vi "nanocal -- nuclear schottky fit V4.vi"() -> ()   [LabVIEW 2020] (continued)
  out "string OUT":string="  \"IDS0158_210310_RAW_cal__ref_\" ->   <| \"ζ\"->  0.331549170129  , \"τ1\"-> 0.031957261989  , \"τS\"-> 0.245155954508  , \"τN\"-> 0.327332604975  , \"τC\"-> 0.001044440547  , \"κ0\"-> 0.000000000511  , \"mm1\"-> 0.000000000000  , \"mm2\"-> 0.000000000000  , \"mm3\"-> 0.000000000000  , \"T\"->  0.140000000000  , \"B\"-> 12.000000000000  , \"θ\"-> 0.000000000000  |>   , \r\"IDS0158_210310_RAW_cal__sam_\" ->   <| \"ζ\"->  0.286336668596  , \"τ1\"-> 0.037477267671  , \"τS\"-> 0.354459287884  , \"τN\"-> 0.444916383639  , \"τC\"-> 0.001225600579  , \"κ0\"-> 0.000000000596  , \"mm1\"-> 0.000000000000  , \"mm2\"-> 0.000000000000  , \"mm3\"-> 0.000000000000  , \"T\"->  0.140000000000  , \"B\"-> 12.000000000000  , \"θ\"-> 0.000000000000  |>   , \r\"IDS0159_210310_RAW_cal__ref_\" ->   <| \"ζ\"->  0.269623663752  , \"τ1\"-> 0.029946823009  , \"τS\"-> 0.193020268264  , \"τN\"-> 0.181925572107  , \"τC\"-> 0.001029221853  , \"κ0\"-> 0.000000000645  , \"mm1\"-> 0.000000000000  , \"mm2\"-> 0.000000000000  , \"mm3\"-> 0.000000000000  , \"T\"->  0.170000000000  , \"B\"-> 12.000000000000  , \"θ\"-> 0.000000000000  |>   , \r\"IDS0159_210310_RAW_cal__sam_\" ->   <| \"ζ\"->  0.219100303741  , \"τ1\"-> 0.028643012604  , \"τS\"-> 0.279362928811  , \"τN\"-> 0.246156444058  , \"τC\"-> 0.001272401549  , \"κ0\"-> 0.000000000760  , \"mm1\"-> 0.000000000000  , \"mm2\"-> 0.000000000000  , \"mm3\"-> 0.000000000000  , \"T\"->  0.170000000000  , \"B\"-> 12.000000000000  , \"θ\"-> 0.000000000000  |>   , \r\"IDS0160_210310_RAW_cal__ref_\" ->   <| \"ζ\"->  0.207047266456  , \"τ1\"-> 0.027475093360  , \"τS\"-> 0.117497913331  , \"τN\"-> 0.102020652890  , \"τC\"-> 0.000950950989  , \"κ0\"-> 0.000000000918  , \"mm1\"-> 0.000000000000  , \"mm2\"-> 0.000000000000  , \"mm3\"-> 0.000000000000  , \"T\"->  0.200000000000  , \"B\"-> 12.000000000000  , \"θ\"-> 0.000000000000  |>   , \r\"IDS0160_210310_RAW_cal__sam_\" ->   <| \"ζ\"->  0.170488637524  , \"τ1\"-> 0.029234231120  , \"τS\"-> 0.149095458227  , \"τN\"-> 0.151792620275  , \"τC\"-> 0.001113424175  , \"κ0\"-> 0.000000001042  , \"mm1\"-> 0.000000000000  , \"mm2\"-> 0.000000000000  , \"mm3\"-> 0.000000000000  , \"T\"->  0.200000000000  , \"B\"-> 12.000000000000  , \"θ\"-> 0.000000000000  |>   , \r\"IDS0161_210310_RAW_cal__ref_\" ->   <| \"ζ\"->  0.165418845287  , \"τ1\"-> 0.025256902580  , \"τS\"-> 0.095232124148  , \"τN\"-> 0.068477414693  , \"τC\"-> 0.001100413424  , \"κ0\"-> 0.000000001058  , \"mm1\"-> 0.000000000000  , \"mm2\"-> 0.000000000000  , \"mm3\"-> 0.000000000000  , \"T\"->  0.220000000000  , \"B\"-> 12.000000000000  , \"θ\"-> 0.000000000000  |>   , \r\"IDS0161_210310_RAW_cal__sam_\" ->   <| \"ζ\"->  0.130531197151  , \"τ1\"-> 0.025704482770  , \"τS\"-> 0.129606657196  , \"τN\"-> 0.091602369165  , \"τC\"-> 0.001441379995  , \"κ0\"-> 0.000000001211  , \"mm1\"-> 0.000000000000  , \"mm2\"-> 0.000000000000  , \"mm3\"-> 0.000000000000  , \"T\"->  0.220000000000  , \"B\"-> 12.000000000000  , \"θ\"-> 0.000000000000  |>   , \r\"IDS0162_210310_RAW_cal__ref_\" ->   <| \"ζ\"->  0.094488415983  , \"τ1\"-> 0.023440091411  , \"τS\"-> 0.070629137621  , \"τN\"-> 0.023695223047  , \"τC\"-> 0.001462465509  , \"κ0\"-> 0.000000001371  , \"mm1\"-> 0.000000000000  , \"mm2\"-> 0.000000000000  , \"mm3\"-> 0.000000000000  , \"T\"->  0.280000000000  , \"B\"-> 12.000000000000  , \"θ\"-> 0.000000000000  |>   , \r\"IDS0162_210310_RAW_cal__sam_\" ->   <| \"ζ\"->  0.078258046754  , \"τ1\"-> 0.028009840731  , \"τS\"-> 0.092122038762  , \"τN\"-> 0.030129595899  , \"τC\"-> 0.001641062244  , \"κ0\"-> 0.000000001543  , \"mm1\"-> 0.000000000000  , \"mm2\"-> 0.000000000000  , \"mm3\"-> 0.000000000000  , \"T\"->  0.280000000000  , \"B\"-> 12.000000000000  , \"θ\"-> 0.000000000000  |>   , \r\"IDS0163_210310_RAW_cal__ref_\" ->   <| \"ζ\"->  0.066045279838  , \"τ1\"-> 0.021690723483  , \"τS\"-> 0.054398710223  , \"τN\"-> 0.012159058060  , \"τC\"-> 0.001677829713  , \"κ0\"-> 0.000000001745  , \"mm1\"-> 0.000000000000  , \"mm2\"-> 0.000000000000  , \"mm3\"-> 0.000000000000  , \"T\"->  0.330000000000  , \"B\"-> 12.000000000000  , \"θ\"-> 0.000000000000  |>   , \r\"IDS0163_210310_RAW_cal__sam_\" ->   <| \"ζ\"->  0.054088186012  , \"τ1\"-> 0.023838802615  , \"τS\"-> 0.069079396629  , \"τN\"-> 0.016435267456  , \"τC\"-> 0.002025071743  , \"κ0\"-> 0.000000001955  , \"mm1\"-> 0.000000000000  , \"mm2\"-> 0.000000000000  , \"mm3\"-> 0.000000000000  , \"T\"->  0.330000000000  , \"B\"-> 12.000000000000  , \"θ\"-> 0.000000000000  |>   , \r\"IDS0164_210310_RAW_cal__ref_\" ->   <| \"ζ\"->  0.046429657722  , \"τ1\"-> 0.021005913305  , \"τS\"-> 0.044250298502  , \"τN\"-> 0.006399419767  , \"τC\"-> 0.002349605146  , \"κ0\"-> 0.000000002166  , \"mm1\"-> 0.000000000000  , \"mm2\"-> 0.000000000000  , \"mm3\"-> 0.000000000000  , \"T\"->  0.400000000000  , \"B\"-> 12.000000000000  , \"θ\"-> 0.000000000000  |>   , \r\"IDS0164_210310_RAW_cal__sam_\" ->   <| \"ζ\"->  0.039314966212  , \"τ1\"-> 0.020712803909  , \"τS\"-> 0.055413767550  , \"τN\"-> 0.008474403424  , \"τC\"-> 0.002674063387  , \"κ0\"-> 0.000000002415  , \"mm1\"-> 0.000000000000  , \"mm2\"-> 0.000000000000  , \"mm3\"-> 0.000000000000  , \"T\"->  0.400000000000  , \"B\"-> 12.000000000000  , \"θ\"-> 0.000000000000  |>   , \r\"IDS0165_210310_RAW_cal__ref_\" ->   <| \"ζ\"->  0.033449822896  , \"τ1\"-> 0.018946770596  , \"τS\"-> 0.035864277160  , \"τN\"-> 0.004007639534  , \"τC\"-> 0.003128970761  , \"κ0\"-> 0.000000002686  , \"mm1\"-> 0.000000000000  , \"mm2\"-> 0.000000000000  , \"mm3\"-> 0.000000000000  , \"T\"->  0.480000000000  , \"B\"-> 12.000000000000  , \"θ\"-> 0.000000000000  |>   , \r\"IDS0165_210310_RAW_cal__sam_\" ->   <| \"ζ\"->  0.031945976845  , \"τ1\"-> 0.019000922826  , \"τS\"-> 0.045624146388  , \"τN\"-> 0.005314716063  , \"τC\"-> 0.002488383471  , \"κ0\"-> 0.000000002954  , \"mm1\"-> 0.000000000000  , \"mm2\"-> 0.000000000000  , \"mm3\"-> 0.000000000000  , \"T\"->  0.480000000000  , \"B\"-> 12.000000000000  , \"θ\"-> 0.000000000000  |>   , \r\"IDS0166_210310_RAW_cal__ref_\" ->   <| \"ζ\"->  0.026131121682  , \"τ1\"-> 0.018837612836  , \"τS\"-> 0.029051745056  , \"τN\"-> 0.002477027845  , \"τC\"-> 0.003638595201  , \"κ0\"-> 0.000000003369  , \"mm1\"-> 0.000000000000  , \"mm2\"-> 0.000000000000  , \"mm3\"-> 0.000000000000  , \"T\"->  0.580000000000  , \"B\"-> 12.000000000000  , \"θ\"-> 0.000000000000  |>   , \r\"IDS0166_210310_RAW_cal__sam_\" ->   <| \"ζ\"->  0.023031239946  , \"τ1\"-> 0.018268814012  , \"τS\"-> 0.037269400776  , \"τN\"-> 0.002696792890  , \"τC\"-> 0.003257395394  , \"κ0\"-> 0.000000003720  , \"mm1\"-> 0.000000000000  , \"mm2\"-> 0.000000000000  , \"mm3\"-> 0.000000000000  , \"T\"->  0.580000000000  , \"B\"-> 12.000000000000  , \"θ\"-> 0.000000000000  |>   , \r\"IDS0167_210310_RAW_cal__ref_\" ->   <| \"ζ\"->  0.026557278794  , \"τ1\"-> 0.016933945977  , \"τS\"-> 0.022881111855  , \"τN\"-> 0.001392473895  , \"τC\"-> 0.004119437148  , \"κ0\"-> 0.000000003981  , \"mm1\"-> 0.000000000000  , \"mm2\"-> 0.000000000000  , \"mm3\"-> 0.000000000000  , \"T\"->  0.680000000000  , \"B\"-> 12.000000000000  , \"θ\"-> 0.000000000000  |>   , \r\"IDS0167_210310_RAW_cal__sam_\" ->   <| \"ζ\"->  0.019920170845  , \"τ1\"-> 0.016368892412  , \"τS\"-> 0.030579536580  , \"τN\"-> 0.001736017565  , \"τC\"-> 0.004971418152  , \"κ0\"-> 0.000000004410  , \"mm1\"-> 0.000000000000  , \"mm2\"-> 0.000000000000  , \"mm3\"-> 0.000000000000  , \"T\"->  0.680000000000  , \"B\"-> 12.000000000000  , \"θ\"-> 0.000000000000  |>   , \r\"IDS0168_210310_RAW_cal__ref_\" ->   <| \"ζ\"->  0.022041296958  , \"τ1\"-> 0.014045615335  , \"τS\"-> 0.018889590451  , \"τN\"-> 0.000813465770  , \"τC\"-> 0.004122617309  , \"κ0\"-> 0.000000005540  , \"mm1\"-> 0.000000000000  , \"mm2\"-> 0.000000000000  , \"mm3\"-> 0.000000000000  , \"T\"->  0.910000000000  , \"B\"-> 12.000000000000  , \"θ\"-> 0.000000000000  |>   , \r\"IDS0168_210310_RAW_cal__sam_\" ->   <| \"ζ\"->  0.017558473054  , \"τ1\"-> 0.014545104284  , \"τS\"-> 0.022979681288  , \"τN\"-> 0.000840829385  , \"τC\"-> 0.005228030240  , \"κ0\"-> 0.000000006068  , \"mm1\"-> 0.000000000000  , \"mm2\"-> 0.000000000000  , \"mm3\"-> 0.000000000000  , \"T\"->  0.910000000000  , \"B\"-> 12.000000000000  , \"θ\"-> 0.000000000000  |>   , \r\"IDS0169_210310_RAW_cal__ref_\" ->   <| \"ζ\"->  0.021090283514  , \"τ1\"-> 0.013945744068  , \"τS\"-> 0.014386606899  , \"τN\"-> 0.000345175874  , \"τC\"-> 0.004902956629  , \"κ0\"-> 0.000000007742  , \"mm1\"-> 0.000000000000  , \"mm2\"-> 0.000000000000  , \"mm3\"-> 0.000000000000  , \"T\"->  1.230000000000  , \"B\"-> 12.000000000000  , \"θ\"-> 0.000000000000  |>   , \r\"IDS0169_210310_RAW_cal__sam_\" ->   <| \"ζ\"->  0.011916480594  , \"τ1\"-> 0.012551282481  , \"τS\"-> 0.018233218660  , \"τN\"-> 0.000345702746  , \"τC\"-> 0.004699451527  , \"κ0\"-> 0.000000008451  , \"mm1\"-> 0.000000000000  , \"mm2\"-> 0.000000000000  , \"mm3\"-> 0.000000000000  , \"T\"->  1.230000000000  , \"B\"-> 12.000000000000  , \"θ\"-> 0.000000000000  |>   , \r\"IDS0170_210310_RAW_cal__ref_\" ->   <| \"ζ\"->  0.021449250230  , \"τ1\"-> 0.014564522147  , \"τS\"-> 0.008878867204  , \"τN\"-> 0.000064984242  , \"τC\"-> 0.006207353748  , \"κ0\"-> 0.000000012530  , \"mm1\"-> 0.000000000000  , \"mm2\"-> 0.000000000000  , \"mm3\"-> 0.000000000000  , \"T\"->  1.970000000000  , \"B\"-> 12.000000000000  , \"θ\"-> 0.000000000000  |>   , \r\"IDS0170_210310_RAW_cal__sam_\" ->   <| \"ζ\"->  0.012831327568  , \"τ1\"-> 0.013315909415  , \"τS\"-> 0.012590836847  , \"τN\"-> 0.000065003013  , \"τC\"-> 0.005276356243  , \"κ0\"-> 0.000000013610  , \"mm1\"-> 0.000000000000  , \"mm2\"-> 0.000000000000  , \"mm3\"-> 0.000000000000  , \"T\"->  1.970000000000  , \"B\"-> 12.000000000000  , \"θ\"-> 0.000000000000  |>   , \r\"IDS0171_210310_RAW_cal__ref_\" ->   <| \"ζ\"->  0.024633693577  , \"τ1\"-> 0.014940694735  , \"τS\"-> 0.006137734482  , \"τN\"-> 0.000014567254  , \"τC\"-> 0.005080683927  , \"κ0\"-> 0.000000022488  , \"mm1\"-> 0.000000000000  , \"mm2\"-> 0.000000000000  , \"mm3\"-> 0.000000000000  , \"T\"->  3.190000000000  , \"B\"-> 12.000000000000  , \"θ\"-> 0.000000000000  |>   , \r\"IDS0171_210310_RAW_cal__sam_\" ->   <| \"ζ\"->  0.019774146838  , \"τ1\"-> 0.013257273421  , \"τS\"-> 0.007064131508  , \"τN\"-> 0.000028000819  , \"τC\"-> 0.006942241845  , \"κ0\"-> 0.000000023477  , \"mm1\"-> 0.000000000000  , \"mm2\"-> 0.000000000000  , \"mm3\"-> 0.000000000000  , \"T\"->  3.190000000000  , \"B\"-> 12.000000000000  , \"θ\"-> 0.000000000000  |>   , \r\"IDS0172_210310_RAW_cal__ref_\" ->   <| \"ζ\"->  0.027835388666  , \"τ1\"-> 0.013976390421  , \"τS\"-> 0.003539188638  , \"τN\"-> 0.000003774856  , \"τC\"-> 0.004420299329  , \"κ0\"-> 0.000000055482  , \"mm1\"-> 0.000000000000  , \"mm2\"-> 0.000000000000  , \"mm3\"-> 0.000000000000  , \"T\"->  5.800000000000  , \"B\"-> 12.000000000000  , \"θ\"-> 0.000000000000  |>   , \r\"IDS0172_210310_RAW_cal__sam_\" ->   <| \"ζ\"->  0.029251354442  , \"τ1\"-> 0.014634751206  , \"τS\"-> 0.003873958746  , \"τN\"-> 0.000007000487  , \"τC\"-> 0.006827504775  , \"κ0\"-> 0.000000056438  , \"mm1\"-> 0.000000000000  , \"mm2\"-> 0.000000000000  , \"mm3\"-> 0.000000000000  , \"T\"->  5.800000000000  , \"B\"-> 12.000000000000  , \"θ\"-> 0.000000000000  |>   , \r\"IDS0181_210310_RAW_cal__ref_\" ->   <| \"ζ\"->  0.194847779603  , \"τ1\"-> 0.071300022200  , \"τS\"-> 0.034370433557  , \"τN\"-> 0.119698958932  , \"τC\"-> 0.001245041457  , \"κ0\"-> 0.000000000909  , \"mm1\"-> 0.000000000000  , \"mm2\"-> 0.000000000000  , \"mm3\"-> 0.000000000000  , \"T\"->  0.179000000000  , \"B\"-> 12.000000000000  , \"θ\"-> 90.000000000000  |>   , \r\"IDS0181_210310_RAW_cal__sam_\" ->   <| \"ζ\"->  0.161975781729  , \"τ1\"-> 0.073089805113  , \"τS\"-> 0.045018408115  , \"τN\"-> 0.161987434028  , \"τC\"-> 0.001482104484  , \"κ0\"-> 0.000000001038  , \"mm1\"-> 0.000000000000  , \"mm2\"-> 0.000000000000  , \"mm3\"-> 0.000000000000  , \"T\"->  0.179000000000  , \"B\"-> 12.000000000000  , \"θ\"-> 90.000000000000  |>   , \r\"IDS0183_210310_RAW_cal__ref_\" ->   <| \"ζ\"->  0.368639553991  , \"τ1\"-> 0.116941860160  , \"τS\"-> 0.051705641175  , \"τN\"-> 0.670097053448  , \"τC\"-> 0.001215131262  , \"κ0\"-> 0.000000000441  , \"mm1\"-> 0.000000000000  , \"mm2\"-> 0.000000000000  , \"mm3\"-> 0.000000000000  , \"T\"->  0.120000000000  , \"B\"-> 12.000000000000  , \"θ\"-> 90.000000000000  |>   , \r\"IDS0183_210310_RAW_cal__sam_\" ->   <| \"ζ\"->  0.300863384227  , \"τ1\"-> 0.104924004009  , \"τS\"-> 0.071070599729  , \"τN\"-> 0.992887187112  , \"τC\"-> 0.001721587800  , \"κ0\"-> 0.000000000548  , \"mm1\"-> 0.000000000000  , \"mm2\"-> 0.000000000000  , \"mm3\"-> 0.000000000000  , \"T\"->  0.120000000000  , \"B\"-> 12.000000000000  , \"θ\"-> 90.000000000000  |>   , \r\"IDS0184_210310_RAW_cal__ref_\" ->   <| \"ζ\"->  0.260731272629  , \"τ1\"-> 0.088447317905  , \"τS\"-> 0.043671964304  , \"τN\"-> 0.254005375090  , \"τC\"-> 0.001151280234  , \"κ0\"-> 0.000000000662  , \"mm1\"-> 0.000000000000  , \"mm2\"-> 0.000000000000  , \"mm3\"-> 0.000000000000  , \"T\"->  0.148000000000  , \"B\"-> 12.000000000000  , \"θ\"-> 90.000000000000  |>   , \r\"IDS0184_210310_RAW_cal__sam_\" ->   <| \"ζ\"->  0.215697702358  , \"τ1\"-> 0.095971807771  , \"τS\"-> 0.069319630290  , \"τN\"-> 0.366712218878  , \"τC\"-> 0.001526252261  , \"κ0\"-> 0.000000000784  , \"mm1\"-> 0.000000000000  , \"mm2\"-> 0.000000000000  , \"mm3\"-> 0.000000000000  , \"T\"->  0.148000000000  , \"B\"-> 12.000000000000  , \"θ\"-> 90.000000000000  |>   , \r\"IDS0185_210310_RAW_cal__ref_\" ->   <| \"ζ\"->  0.166318035375  , \"τ1\"-> 0.066119695107  , \"τS\"-> 0.031891479777  , \"τN\"-> 0.088107606578  , \"τC\"-> 0.001299933301  , \"κ0\"-> 0.000000001075  , \"mm1\"-> 0.000000000000  , \"mm2\"-> 0.000000000000  , \"mm3\"-> 0.000000000000  , \"T\"->  0.197000000000  , \"B\"-> 12.000000000000  , \"θ\"-> 90.000000000000  |>   , \r\"IDS0185_210310_RAW_cal__sam_\" ->   <| \"ζ\"->  0.139117463690  , \"τ1\"-> 0.070330410174  , \"τS\"-> 0.040829719954  , \"τN\"-> 0.122434321115  , \"τC\"-> 0.001436112939  , \"κ0\"-> 0.000000001208  , \"mm1\"-> 0.000000000000  , \"mm2\"-> 0.000000000000  , \"mm3\"-> 0.000000000000  , \"T\"->  0.197000000000  , \"B\"-> 12.000000000000  , \"θ\"-> 90.000000000000  |>   , \r\"IDS0186_210310_RAW_cal__ref_\" ->   <| \"ζ\"->  0.101265410351  , \"τ1\"-> 0.051590946451  , \"τS\"-> 0.026920044229  , \"τN\"-> 0.035536954174  , \"τC\"-> 0.001490330879  , \"κ0\"-> 0.000000001364  , \"mm1\"-> 0.000000000000  , \"mm2\"-> 0.000000000000  , \"mm3\"-> 0.000000000000  , \"T\"->  0.249000000000  , \"B\"-> 12.000000000000  , \"θ\"-> 90.000000000000  |>   , \r\"IDS0186_210310_RAW_cal__sam_\" ->   <| \"ζ\"->  0.079912790251  , \"τ1\"-> 0.053932962768  , \"τS\"-> 0.033847624645  , \"τN\"-> 0.047947649984  , \"τC\"-> 0.001828917906  , \"κ0\"-> 0.000000001546  , \"mm1\"-> 0.000000000000  , \"mm2\"-> 0.000000000000  , \"mm3\"-> 0.000000000000  , \"T\"->  0.249000000000  , \"B\"-> 12.000000000000  , \"θ\"-> 90.000000000000  |>   , \r\"IDS0187_210310_RAW_cal__ref_\" ->   <| \"ζ\"->  0.070401604603  , \"τ1\"-> 0.043684283216  , \"τS\"-> 0.023756676354  , \"τN\"-> 0.017570167589  , \"τC\"-> 0.001809460237  , \"κ0\"-> 0.000000001742  , \"mm1\"-> 0.000000000000  , \"mm2\"-> 0.000000000000  , \"mm3\"-> 0.000000000000  , \"T\"->  0.300000000000  , \"B\"-> 12.000000000000  , \"θ\"-> 90.000000000000  |>   , \r\"IDS0187_210310_RAW_cal__sam_\" ->   <| \"ζ\"->  0.057938569833  , \"τ1\"-> 0.045244527663  , \"τS\"-> 0.029709028064  , \"τN\"-> 0.023577376257  , \"τC\"-> 0.002006607539  , \"κ0\"-> 0.000000001948  , \"mm1\"-> 0.000000000000  , \"mm2\"-> 0.000000000000  , \"mm3\"-> 0.000000000000  , \"T\"->  0.300000000000  , \"B\"-> 12.000000000000  , \"θ\"-> 90.000000000000  |>   , \r\"IDS0188_210310_RAW_cal__ref_\" ->   <| \"ζ\"->  0.052039078112  , \"τ1\"-> 0.037833987996  , \"τS\"-> 0.021664376950  , \"τN\"-> 0.010364100672  , \"τC\"-> 0.002302914949  , \"κ0\"-> 0.000000002119  , \"mm1\"-> 0.000000000000  , \"mm2\"-> 0.000000000000  , \"mm3\"-> 0.000000000000  , \"T\"->  0.360000000000  , \"B\"-> 12.000000000000  , \"θ\"-> 90.000000000000  |>   , \r\"IDS0188_210310_RAW_cal__sam_\" ->   <| \"ζ\"->  0.044154556051  , \"τ1\"-> 0.038823125235  , \"τS\"-> 0.027069314930  , \"τN\"-> 0.013601990730  , \"τC\"-> 0.002287979276  , \"κ0\"-> 0.000000002359  , \"mm1\"-> 0.000000000000  , \"mm2\"-> 0.000000000000  , \"mm3\"-> 0.000000000000  , \"T\"->  0.360000000000  , \"B\"-> 12.000000000000  , \"θ\"-> 90.000000000000  |>   , \r\"IDS0189_210310_RAW_cal__ref_\" ->   <| \"ζ\"->  0.040584680050  , \"τ1\"-> 0.030359591877  , \"τS\"-> 0.019792901852  , \"τN\"-> 0.005324821183  , \"τC\"-> 0.002700986774  , \"κ0\"-> 0.000000002671  , \"mm1\"-> 0.000000000000  , \"mm2\"-> 0.000000000000  , \"mm3\"-> 0.000000000000  , \"T\"->  0.430000000000  , \"B\"-> 12.000000000000  , \"θ\"-> 90.000000000000  |>   , \r\"IDS0189_210310_RAW_cal__sam_\" ->   <| \"ζ\"->  0.032748569996  , \"τ1\"-> 0.031072007290  , \"τS\"-> 0.024343937548  , \"τN\"-> 0.006961654481  , \"τC\"-> 0.002967111565  , \"κ0\"-> 0.000000002964  , \"mm1\"-> 0.000000000000  , \"mm2\"-> 0.000000000000  , \"mm3\"-> 0.000000000000  , \"T\"->  0.430000000000  , \"B\"-> 12.000000000000  , \"θ\"-> 90.000000000000  |>   , \r\"IDS0190_210310_RAW_cal__ref_\" ->   <| \"ζ\"->  0.030700897923  , \"τ1\"-> 0.026935085078  , \"τS\"-> 0.018364864329  , \"τN\"-> 0.002898516959  , \"τC\"-> 0.003150649099  , \"κ0\"-> 0.000000003342  , \"mm1\"-> 0.000000000000  , \"mm2\"-> 0.000000000000  , \"mm3\"-> 0.000000000000  , \"T\"->  0.512000000000  , \"B\"-> 12.000000000000  , \"θ\"-> 90.000000000000  |>   , \r\"IDS0190_210310_RAW_cal__sam_\" ->   <| \"ζ\"->  0.027599263457  , \"τ1\"-> 0.026239105728  , \"τS\"-> 0.022370859308  , \"τN\"-> 0.003857632966  , \"τC\"-> 0.003499360499  , \"κ0\"-> 0.000000003681  , \"mm1\"-> 0.000000000000  , \"mm2\"-> 0.000000000000  , \"mm3\"-> 0.000000000000  , \"T\"->  0.512000000000  , \"B\"-> 12.000000000000  , \"θ\"-> 90.000000000000  |>   , \r\"IDS0191_210310_RAW_cal__ref_\" ->   <| \"ζ\"->  0.025322625458  , \"τ1\"-> 0.023401812401  , \"τS\"-> 0.017347416709  , \"τN\"-> 0.002020498851  , \"τC\"-> 0.003594259467  , \"κ0\"-> 0.000000003970  , \"mm1\"-> 0.000000000000  , \"mm2\"-> 0.000000000000  , \"mm3\"-> 0.000000000000  , \"T\"->  0.610000000000  , \"B\"-> 12.000000000000  , \"θ\"-> 90.000000000000  |>   , \r\"IDS0191_210310_RAW_cal__sam_\" ->   <| \"ζ\"->  0.020568815513  , \"τ1\"-> 0.023045965648  , \"τS\"-> 0.020791387386  , \"τN\"-> 0.002229171297  , \"τC\"-> 0.004427475438  , \"κ0\"-> 0.000000004398  , \"mm1\"-> 0.000000000000  , \"mm2\"-> 0.000000000000  , \"mm3\"-> 0.000000000000  , \"T\"->  0.610000000000  , \"B\"-> 12.000000000000  , \"θ\"-> 90.000000000000  |>   , \r\"IDS0192_210310_RAW_cal__ref_\" ->   <| \"ζ\"->  0.022100596026  , \"τ1\"-> 0.020519097823  , \"τS\"-> 0.015555141042  , \"τN\"-> 0.000889956832  , \"τC\"-> 0.004354791503  , \"κ0\"-> 0.000000005560  , \"mm1\"-> 0.000000000000  , \"mm2\"-> 0.000000000000  , \"mm3\"-> 0.000000000000  , \"T\"->  0.810000000000  , \"B\"-> 12.000000000000  , \"θ\"-> 90.000000000000  |>   , \r\"IDS0192_210310_RAW_cal__sam_\" ->   <| \"ζ\"->  0.016548170999  , \"τ1\"-> 0.020108887890  , \"τS\"-> 0.018558394948  , \"τN\"-> 0.001160732495  , \"τC\"-> 0.004746126241  , \"κ0\"-> 0.000000005882  , \"mm1\"-> 0.000000000000  , \"mm2\"-> 0.000000000000  , \"mm3\"-> 0.000000000000  , \"T\"->  0.810000000000  , \"B\"-> 12.000000000000  , \"θ\"-> 90.000000000000  |>   , \r\"IDS0193_210310_RAW_cal__ref_\" ->   <| \"ζ\"->  0.020969814378  , \"τ1\"-> 0.020016820130  , \"τS\"-> 0.013372894745  , \"τN\"-> 0.000454586591  , \"τC\"-> 0.005292751338  , \"κ0\"-> 0.000000007771  , \"mm1\"-> 0.000000000000  , \"mm2\"-> 0.000000000000  , \"mm3\"-> 0.000000000000  , \"T\"->  1.100000000000  , \"B\"-> 12.000000000000  , \"θ\"-> 90.000000000000  |>   , \r\"IDS0193_210310_RAW_cal__sam_\" ->   <| \"ζ\"->  0.014495870556  , \"τ1\"-> 0.019990087457  , \"τS\"-> 0.016832201384  , \"τN\"-> 0.000455517238  , \"τC\"-> 0.005555782498  , \"κ0\"-> 0.000000008420  , \"mm1\"-> 0.000000000000  , \"mm2\"-> 0.000000000000  , \"mm3\"-> 0.000000000000  , \"T\"->  1.100000000000  , \"B\"-> 12.000000000000  , \"θ\"-> 90.000000000000  |>   , \r\"IDS0194_210310_RAW_cal__ref_\" ->   <| \"ζ\"->  0.020900896759  , \"τ1\"-> 0.018288874472  , \"τS\"-> 0.009095511262  , \"τN\"-> 0.000107884456  , \"τC\"-> 0.006896232004  , \"κ0\"-> 0.000000013449  , \"mm1\"-> 0.000000000000  , \"mm2\"-> 0.000000000000  , \"mm3\"-> 0.000000000000  , \"T\"->  1.800000000000  , \"B\"-> 12.000000000000  , \"θ\"-> 90.000000000000  |>   , \r\"IDS0194_210310_RAW_cal__sam_\" ->   <| \"ζ\"->  0.014043763709  , \"τ1\"-> 0.018292068543  , \"τS\"-> 0.011311396743  , \"τN\"-> 0.000128802259  , \"τC\"-> 0.008087849636  , \"κ0\"-> 0.000000014258  , \"mm1\"-> 0.000000000000  , \"mm2\"-> 0.000000000000  , \"mm3\"-> 0.000000000000  , \"T\"->  1.800000000000  , \"B\"-> 12.000000000000  , \"θ\"-> 90.000000000000  |>   , \r\"IDS0195_210310_RAW_cal__ref_\" ->   <| \"ζ\"->  0.019765118173  , \"τ1\"-> 0.018324978618  , \"τS\"-> 0.006054329354  , \"τN\"-> 0.000028420666  , \"τC\"-> 0.006398306925  , \"κ0\"-> 0.000000023958  , \"mm1\"-> 0.000000000000  , \"mm2\"-> 0.000000000000  , \"mm3\"-> 0.000000000000  , \"T\"->  3.000000000000  , \"B\"-> 12.000000000000  , \"θ\"-> 90.000000000000  |>   , \r\"IDS0195_210310_RAW_cal__sam_\" ->   <| \"ζ\"->  0.016187684631  , \"τ1\"-> 0.018325345271  , \"τS\"-> 0.007510087776  , \"τN\"-> 0.000028419157  , \"τC\"-> 0.008115463080  , \"κ0\"-> 0.000000024747  , \"mm1\"-> 0.000000000000  , \"mm2\"-> 0.000000000000  , \"mm3\"-> 0.000000000000  , \"T\"->  3.000000000000  , \"B\"-> 12.000000000000  , \"θ\"-> 90.000000000000  |>   , \r\"IDS0196_210310_RAW_cal__ref_\" ->   <| \"ζ\"->  0.030164668817  , \"τ1\"-> 0.012822215558  , \"τS\"-> 0.004108197943  , \"τN\"-> 0.000006999504  , \"τC\"-> 0.004420975765  , \"κ0\"-> 0.000000058872  , \"mm1\"-> 0.000000000000  , \"mm2\"-> 0.000000000000  , \"mm3\"-> 0.000000000000  , \"T\"->  5.700000000000  , \"B\"-> 12.000000000000  , \"θ\"-> 90.000000000000  |>   , \r\"IDS0196_210310_RAW_cal__sam_\" ->   <| \"ζ\"->  0.027897403691  , \"τ1\"-> 0.014639690770  , \"τS\"-> 0.004105291179  , \"τN\"-> 0.000006999171  , \"τC\"-> 0.007414449545  , \"κ0\"-> 0.000000059701  , \"mm1\"-> 0.000000000000  , \"mm2\"-> 0.000000000000  , \"mm3\"-> 0.000000000000  , \"T\"->  5.700000000000  , \"B\"-> 12.000000000000  , \"θ\"-> 90.000000000000  |>   , \r\"IDS0208_210310_RAW_cal__ref_\" ->   <| \"ζ\"->  0.000000000000  , \"τ1\"-> 0.000000000000  , \"τS\"-> 0.000000000000  , \"τN\"-> 0.000000000000  , \"τC\"-> 0.000000000000  , \"κ0\"-> 0.000000000000  , \"mm1\"-> 0.000000000000  , \"mm2\"-> 0.000000000000  , \"mm3\"-> 0.000000000000  , \"T\"->  0.197000000000  , \"B\"-> 0.000000000000  , \"θ\"-> 0.000000000000  |>   , \r\"IDS0208_210310_RAW_cal__sam_\" ->   <| \"ζ\"->  0.000000000000  , \"τ1\"-> 0.000000000000  , \"τS\"-> 0.000000000000  , \"τN\"-> 0.000000000000  , \"τC\"-> 0.000000000000  , \"κ0\"-> 0.000000000000  , \"mm1\"-> 0.000000000000  , \"mm2\"-> 0.000000000000  , \"mm3\"-> 0.000000000000  , \"T\"->  0.197000000000  , \"B\"-> 0.000000000000  , \"θ\"-> 0.000000000000  |>   , \r\"IDS0209_210310_RAW_cal__ref_\" ->   <| \"ζ\"->  0.163571654798  , \"τ1\"-> 0.020520714675  , \"τS\"-> 0.073117323271  , \"τN\"-> 0.020627224399  , \"τC\"-> 0.001336341391  , \"κ0\"-> 0.000000001061  , \"mm1\"-> 0.000000000000  , \"mm2\"-> 0.000000000000  , \"mm3\"-> 0.000000000000  , \"T\"->  0.197000000000  , \"B\"-> 0.000000000000  , \"θ\"-> 0.000000000000  |>   , \r\"IDS0209_210310_RAW_cal__sam_\" ->   <| \"ζ\"->  0.132901556203  , \"τ1\"-> 0.022795175616  , \"τS\"-> 0.082481385864  , \"τN\"-> 0.041432545456  , \"τC\"-> 0.001408424074  , \"κ0\"-> 0.000000001182  , \"mm1\"-> 0.000000000000  , \"mm2\"-> 0.000000000000  , \"mm3\"-> 0.000000000000  , \"T\"->  0.197000000000  , \"B\"-> 0.000000000000  , \"θ\"-> 0.000000000000  |>   , \r\"IDS0210_210310_RAW_cal__ref_\" ->   <| \"ζ\"->  0.000000000000  , \"τ1\"-> 0.000000000000  , \"τS\"-> 0.000000000000  , \"τN\"-> 0.000000000000  , \"τC\"-> 0.000000000000  , \"κ0\"-> 0.000000000000  , \"mm1\"-> 0.000000000000  , \"mm2\"-> 0.000000000000  , \"mm3\"-> 0.000000000000  , \"T\"->  0.148000000000  , \"B\"-> 6.000000000000  , \"θ\"-> 0.000000000000  |>   , \r\"IDS0210_210310_RAW_cal__sam_\" ->   <| \"ζ\"->  0.000000000000  , \"τ1\"-> 0.000000000000  , \"τS\"-> 0.000000000000  , \"τN\"-> 0.000000000000  , \"τC\"-> 0.000000000000  , \"κ0\"-> 0.000000000000  , \"mm1\"-> 0.000000000000  , \"mm2\"-> 0.000000000000  , \"mm3\"-> 0.000000000000  , \"T\"->  0.148000000000  , \"B\"-> 6.000000000000  , \"θ\"-> 0.000000000000  |>   , \r\"IDS0211_210310_RAW_cal__ref_\" ->   <| \"ζ\"->  0.160882265826  , \"τ1\"-> 0.034919932965  , \"τS\"-> 0.043973777096  , \"τN\"-> 0.047289018614  , \"τC\"-> 0.001339652100  , \"κ0\"-> 0.000000001069  , \"mm1\"-> 0.000000000000  , \"mm2\"-> 0.000000000000  , \"mm3\"-> 0.000000000000  , \"T\"->  0.197000000000  , \"B\"-> 9.000000000000  , \"θ\"-> 0.000000000000  |>   , \r\"IDS0211_210310_RAW_cal__sam_\" ->   <| \"ζ\"->  0.132534999612  , \"τ1\"-> 0.042581417401  , \"τS\"-> 0.054103824371  , \"τN\"-> 0.072163013930  , \"τC\"-> 0.001421040158  , \"κ0\"-> 0.000000001190  , \"mm1\"-> 0.000000000000  , \"mm2\"-> 0.000000000000  , \"mm3\"-> 0.000000000000  , \"T\"->  0.197000000000  , \"B\"-> 9.000000000000  , \"θ\"-> 0.000000000000  |>   , \r\"IDS0212_210310_RAW_cal__ref_\" ->   <| \"ζ\"->  0.154351103049  , \"τ1\"-> 0.051844552801  , \"τS\"-> 0.034651211615  , \"τN\"-> 0.065884588100  , \"τC\"-> 0.001166375427  , \"κ0\"-> 0.000000001084  , \"mm1\"-> 0.000000000000  , \"mm2\"-> 0.000000000000  , \"mm3\"-> 0.000000000000  , \"T\"->  0.197000000000  , \"B\"-> 11.000000000000  , \"θ\"-> 0.000000000000  |>   , \r\"IDS0212_210310_RAW_cal__sam_\" ->   <| \"ζ\"->  0.124414912597  , \"τ1\"-> 0.052685716706  , \"τS\"-> 0.041788480794  , \"τN\"-> 0.092820346766  , \"τC\"-> 0.001183564004  , \"κ0\"-> 0.000000001217  , \"mm1\"-> 0.000000000000  , \"mm2\"-> 0.000000000000  , \"mm3\"-> 0.000000000000  , \"T\"->  0.197000000000  , \"B\"-> 11.000000000000  , \"θ\"-> 0.000000000000  |>   , \r\"IDS0213_210310_RAW_cal__ref_\" ->   <| \"ζ\"->  0.158514180755  , \"τ1\"-> 0.046388884826  , \"τS\"-> 0.038847986012  , \"τN\"-> 0.058494864948  , \"τC\"-> 0.001325817289  , \"κ0\"-> 0.000000001072  , \"mm1\"-> 0.000000000000  , \"mm2\"-> 0.000000000000  , \"mm3\"-> 0.000000000000  , \"T\"->  0.197000000000  , \"B\"-> 10.000000000000  , \"θ\"-> 0.000000000000  |>   , \r\"IDS0213_210310_RAW_cal__sam_\" ->   <| \"ζ\"->  0.130083148284  , \"τ1\"-> 0.046211117525  , \"τS\"-> 0.046173592526  , \"τN\"-> 0.081942172735  , \"τC\"-> 0.001380184863  , \"κ0\"-> 0.000000001209  , \"mm1\"-> 0.000000000000  , \"mm2\"-> 0.000000000000  , \"mm3\"-> 0.000000000000  , \"T\"->  0.197000000000  , \"B\"-> 10.000000000000  , \"θ\"-> 0.000000000000  |>   , \r\"IDS0214_210310_RAW_cal__ref_\" ->   <| \"ζ\"->  0.154362032240  , \"τ1\"-> 0.030258273194  , \"τS\"-> 0.049523350330  , \"τN\"-> 0.040015703513  , \"τC\"-> 0.001328953616  , \"κ0\"-> 0.000000001075  , \"mm1\"-> 0.000000000000  , \"mm2\"-> 0.000000000000  , \"mm3\"-> 0.000000000000  , \"T\"->  0.197000000000  , \"B\"-> 8.000000000000  , \"θ\"-> 0.000000000000  |>   , \r\"IDS0214_210310_RAW_cal__sam_\" ->   <| \"ζ\"->  0.126440702434  , \"τ1\"-> 0.034118036572  , \"τS\"-> 0.060921114440  , \"τN\"-> 0.059832148427  , \"τC\"-> 0.001404471084  , \"κ0\"-> 0.000000001199  , \"mm1\"-> 0.000000000000  , \"mm2\"-> 0.000000000000  , \"mm3\"-> 0.000000000000  , \"T\"->  0.197000000000  , \"B\"-> 8.000000000000  , \"θ\"-> 0.000000000000  |>   , \r\"IDS0215_210310_RAW_cal__ref_\" ->   <| \"ζ\"->  0.162645417184  , \"τ1\"-> 0.023693851446  , \"τS\"-> 0.062400062170  , \"τN\"-> 0.026326088223  , \"τC\"-> 0.001322053294  , \"κ0\"-> 0.000000001070  , \"mm1\"-> 0.000000000000  , \"mm2\"-> 0.000000000000  , \"mm3\"-> 0.000000000000  , \"T\"->  0.197000000000  , \"B\"-> 7.000000000000  , \"θ\"-> 0.000000000000  |>   , \r\"IDS0215_210310_RAW_cal__sam_\" ->   <| \"ζ\"->  0.131383255045  , \"τ1\"-> 0.026827335842  , \"τS\"-> 0.071725959535  , \"τN\"-> 0.047510049318  , \"τC\"-> 0.001407613780  , \"κ0\"-> 0.000000001187  , \"mm1\"-> 0.000000000000  , \"mm2\"-> 0.000000000000  , \"mm3\"-> 0.000000000000  , \"T\"->  0.197000000000  , \"B\"-> 7.000000000000  , \"θ\"-> 0.000000000000  |>   , \r\"IDS0216_210310_RAW_cal__ref_\" ->   <| \"ζ\"->  0.149904026692  , \"τ1\"-> 0.020347243982  , \"τS\"-> 0.075273674904  , \"τN\"-> 0.020640082408  , \"τC\"-> 0.001432916876  , \"κ0\"-> 0.000000001050  , \"mm1\"-> 0.000000000000  , \"mm2\"-> 0.000000000000  , \"mm3\"-> 0.000000000000  , \"T\"->  0.197000000000  , \"B\"-> 5.000000000000  , \"θ\"-> 0.000000000000  |>   , \r\"IDS0216_210310_RAW_cal__sam_\" ->   <| \"ζ\"->  0.125455081262  , \"τ1\"-> 0.021777951907  , \"τS\"-> 0.089086097551  , \"τN\"-> 0.033580911935  , \"τC\"-> 0.001437991682  , \"κ0\"-> 0.000000001167  , \"mm1\"-> 0.000000000000  , \"mm2\"-> 0.000000000000  , \"mm3\"-> 0.000000000000  , \"T\"->  0.197000000000  , \"B\"-> 5.000000000000  , \"θ\"-> 0.000000000000  |>   , \r\"IDS0217_210310_RAW_cal__ref_\" ->   <| \"ζ\"->  0.121305227705  , \"τ1\"-> 0.032098202143  , \"τS\"-> 0.011865067519  , \"τN\"-> 0.005878702730  , \"τC\"-> 0.002147559783  , \"κ0\"-> 0.000000001032  , \"mm1\"-> 0.000000000000  , \"mm2\"-> 0.000000000000  , \"mm3\"-> 0.000000000000  , \"T\"->  0.197000000000  , \"B\"-> 0.000000000000  , \"θ\"-> 0.000000000000  |>   , \r\"IDS0217_210310_RAW_cal__sam_\" ->   <| \"ζ\"->  0.101804363109  , \"τ1\"-> 0.031947692776  , \"τS\"-> 0.014125667853  , \"τN\"-> 0.006009042128  , \"τC\"-> 0.002323789932  , \"κ0\"-> 0.000000001168  , \"mm1\"-> 0.000000000000  , \"mm2\"-> 0.000000000000  , \"mm3\"-> 0.000000000000  , \"T\"->  0.197000000000  , \"B\"-> 0.000000000000  , \"θ\"-> 0.000000000000  |>   , \r\"IDS0218_210310_RAW_cal__ref_\" ->   <| \"ζ\"->  0.000000000000  , \"τ1\"-> 0.000000000000  , \"τS\"-> 0.000000000000  , \"τN\"-> 0.000000000000  , \"τC\"-> 0.000000000000  , \"κ0\"-> 0.000000000000  , \"mm1\"-> 0.000000000000  , \"mm2\"-> 0.000000000000  , \"mm3\"-> 0.000000000000  , \"T\"->  1.550000000000  , \"B\"-> 0.000000000000  , \"θ\"-> 0.000000000000  |>   , \r\"IDS0218_210310_RAW_cal__sam_\" ->   <| \"ζ\"->  0.000000000000  , \"τ1\"-> 0.000000000000  , \"τS\"-> 0.000000000000  , \"τN\"-> 0.000000000000  , \"τC\"-> 0.000000000000  , \"κ0\"-> 0.000000000000  , \"mm1\"-> 0.000000000000  , \"mm2\"-> 0.000000000000  , \"mm3\"-> 0.000000000000  , \"T\"->  1.550000000000  , \"B\"-> 0.000000000000  , \"θ\"-> 0.000000000000  |>   , \r\"IDS0219_210310_RAW_cal__ref_\" ->   <| \"ζ\"->  0.000000000000  , \"τ1\"-> 0.000000000000  , \"τS\"-> 0.000000000000  , \"τN\"-> 0.000000000000  , \"τC\"-> 0.000000000000  , \"κ0\"-> 0.000000000000  , \"mm1\"-> 0.000000000000  , \"mm2\"-> 0.000000000000  , \"mm3\"-> 0.000000000000  , \"T\"->  1.000000000000  , \"B\"-> 0.000000000000  , \"θ\"-> 0.000000000000  |>   , \r\"IDS0219_210310_RAW_cal__sam_\" ->   <| \"ζ\"->  0.000000000000  , \"τ1\"-> 0.000000000000  , \"τS\"-> 0.000000000000  , \"τN\"-> 0.000000000000  , \"τC\"-> 0.000000000000  , \"κ0\"-> 0.000000000000  , \"mm1\"-> 0.000000000000  , \"mm2\"-> 0.000000000000  , \"mm3\"-> 0.000000000000  , \"T\"->  1.000000000000  , \"B\"-> 0.000000000000  , \"θ\"-> 0.000000000000  |>   , \r\"IDS0220_210310_RAW_cal__ref_\" ->   <| \"ζ\"->  0.000000000000  , \"τ1\"-> 0.000000000000  , \"τS\"-> 0.000000000000  , \"τN\"-> 0.000000000000  , \"τC\"-> 0.000000000000  , \"κ0\"-> 0.000000000000  , \"mm1\"-> 0.000000000000  , \"mm2\"-> 0.000000000000  , \"mm3\"-> 0.000000000000  , \"T\"->  0.677000000000  , \"B\"-> 0.000000000000  , \"θ\"-> 0.000000000000  |>   , \r\"IDS0220_210310_RAW_cal__sam_\" ->   <| \"ζ\"->  0.000000000000  , \"τ1\"-> 0.000000000000  , \"τS\"-> 0.000000000000  , \"τN\"-> 0.000000000000  , \"τC\"-> 0.000000000000  , \"κ0\"-> 0.000000000000  , \"mm1\"-> 0.000000000000  , \"mm2\"-> 0.000000000000  , \"mm3\"-> 0.000000000000  , \"T\"->  0.677000000000  , \"B\"-> 0.000000000000  , \"θ\"-> 0.000000000000  |>   , \r\"IDS0224_210310_RAW_cal__ref_\" ->   <| \"ζ\"->  0.000000000000  , \"τ1\"-> 0.000000000000  , \"τS\"-> 0.000000000000  , \"τN\"-> 0.000000000000  , \"τC\"-> 0.000000000000  , \"κ0\"-> 0.000000000000  , \"mm1\"-> 0.000000000000  , \"mm2\"-> 0.000000000000  , \"mm3\"-> 0.000000000000  , \"T\"->  0.000000000000  , \"B\"-> 0.000000000000  , \"θ\"-> 0.000000000000  |>   , \r\"IDS0224_210310_RAW_cal__sam_\" ->   <| \"ζ\"->  0.000000000000  , \"τ1\"-> 0.000000000000  , \"τS\"-> 0.000000000000  , \"τN\"-> 0.000000000000  , \"τC\"-> 0.000000000000  , \"κ0\"-> 0.000000000000  , \"mm1\"-> 0.000000000000  , \"mm2\"-> 0.000000000000  , \"mm3\"-> 0.000000000000  , \"T\"->  0.000000000000  , \"B\"-> 0.000000000000  , \"θ\"-> 0.000000000000  |>   , \r\"IDS0293_210427_RAW_cal__ref_\" ->   <| \"ζ\"->  0.016384838586  , \"τ1\"-> 0.013784349529  , \"τS\"-> 0.011495286759  , \"τN\"-> 0.000117117954  , \"τC\"-> 0.004048153799  , \"κ0\"-> 0.000000013122  , \"mm1\"-> 0.000000000000  , \"mm2\"-> 0.000000000000  , \"mm3\"-> 0.000000000000  , \"T\"->  1.900000000000  , \"B\"-> 12.000000000000  , \"θ\"-> 30.000000000000  |>   , \r\"IDS0293_210427_RAW_cal__sam_\" ->   <| \"ζ\"->  0.009772435939  , \"τ1\"-> 0.020827345370  , \"τS\"-> 0.013809334085  , \"τN\"-> 0.000168485133  , \"τC\"-> 0.005555066716  , \"κ0\"-> 0.000000013930  , \"mm1\"-> 0.000000000000  , \"mm2\"-> 0.000000000000  , \"mm3\"-> 0.000000000000  , \"T\"->  1.900000000000  , \"B\"-> 12.000000000000  , \"θ\"-> 30.000000000000  |>   , \r\"IDS0294_210427_RAW_cal__ref_\" ->   <| \"ζ\"->  0.017975147456  , \"τ1\"-> 0.015573317032  , \"τS\"-> 0.016697357463  , \"τN\"-> 0.000401487663  , \"τC\"-> 0.004243374884  , \"κ0\"-> 0.000000007622  , \"mm1\"-> 0.000000000000  , \"mm2\"-> 0.000000000000  , \"mm3\"-> 0.000000000000  , \"T\"->  1.130000000000  , \"B\"-> 12.000000000000  , \"θ\"-> 30.000000000000  |>   , \r\"IDS0294_210427_RAW_cal__sam_\" ->   <| \"ζ\"->  0.010912011148  , \"τ1\"-> 0.020760977312  , \"τS\"-> 0.021106239637  , \"τN\"-> 0.000452316988  , \"τC\"-> 0.005003723454  , \"κ0\"-> 0.000000008194  , \"mm1\"-> 0.000000000000  , \"mm2\"-> 0.000000000000  , \"mm3\"-> 0.000000000000  , \"T\"->  1.130000000000  , \"B\"-> 12.000000000000  , \"θ\"-> 30.000000000000  |>   , \r\"IDS0295_210427_RAW_cal__ref_\" ->   <| \"ζ\"->  0.021360373560  , \"τ1\"-> 0.017226807214  , \"τS\"-> 0.021136224671  , \"τN\"-> 0.000857882935  , \"τC\"-> 0.004088468956  , \"κ0\"-> 0.000000005432  , \"mm1\"-> 0.000000000000  , \"mm2\"-> 0.000000000000  , \"mm3\"-> 0.000000000000  , \"T\"->  0.830000000000  , \"B\"-> 12.000000000000  , \"θ\"-> 30.000000000000  |>   , \r\"IDS0295_210427_RAW_cal__sam_\" ->   <| \"ζ\"->  0.013460153434  , \"τ1\"-> 0.020684726260  , \"τS\"-> 0.027140346721  , \"τN\"-> 0.000960302406  , \"τC\"-> 0.004517434882  , \"κ0\"-> 0.000000005889  , \"mm1\"-> 0.000000000000  , \"mm2\"-> 0.000000000000  , \"mm3\"-> 0.000000000000  , \"T\"->  0.830000000000  , \"B\"-> 12.000000000000  , \"θ\"-> 30.000000000000  |>   , \r\"IDS0296_210427_RAW_cal__ref_\" ->   <| \"ζ\"->  0.027756025784  , \"τ1\"-> 0.019742757718  , \"τS\"-> 0.026611973171  , \"τN\"-> 0.001398943183  , \"τC\"-> 0.003482574473  , \"κ0\"-> 0.000000003907  , \"mm1\"-> 0.000000000000  , \"mm2\"-> 0.000000000000  , \"mm3\"-> 0.000000000000  , \"T\"->  0.620000000000  , \"B\"-> 12.000000000000  , \"θ\"-> 30.000000000000  |>   , \r\"IDS0296_210427_RAW_cal__sam_\" ->   <| \"ζ\"->  0.016892016292  , \"τ1\"-> 0.020344757415  , \"τS\"-> 0.033845756966  , \"τN\"-> 0.001946817417  , \"τC\"-> 0.004013762913  , \"κ0\"-> 0.000000004252  , \"mm1\"-> 0.000000000000  , \"mm2\"-> 0.000000000000  , \"mm3\"-> 0.000000000000  , \"T\"->  0.620000000000  , \"B\"-> 12.000000000000  , \"θ\"-> 30.000000000000  |>   , \r\"IDS0297_210427_RAW_cal__ref_\" ->   <| \"ζ\"->  0.034775017342  , \"τ1\"-> 0.018923965005  , \"τS\"-> 0.030086686370  , \"τN\"-> 0.002286572055  , \"τC\"-> 0.002714831651  , \"κ0\"-> 0.000000003294  , \"mm1\"-> 0.000000000000  , \"mm2\"-> 0.000000000000  , \"mm3\"-> 0.000000000000  , \"T\"->  0.530000000000  , \"B\"-> 12.000000000000  , \"θ\"-> 30.000000000000  |>   , \r\"IDS0297_210427_RAW_cal__sam_\" ->   <| \"ζ\"->  0.021116250068  , \"τ1\"-> 0.020669239851  , \"τS\"-> 0.037941648749  , \"τN\"-> 0.003221866945  , \"τC\"-> 0.003619427775  , \"κ0\"-> 0.000000003553  , \"mm1\"-> 0.000000000000  , \"mm2\"-> 0.000000000000  , \"mm3\"-> 0.000000000000  , \"T\"->  0.530000000000  , \"B\"-> 12.000000000000  , \"θ\"-> 30.000000000000  |>   , \r\"IDS0298_210427_RAW_cal__ref_\" ->   <| \"ζ\"->  0.046396907778  , \"τ1\"-> 0.018912834926  , \"τS\"-> 0.034035556993  , \"τN\"-> 0.004466176128  , \"τC\"-> 0.002290347128  , \"κ0\"-> 0.000000002639  , \"mm1\"-> 0.000000000000  , \"mm2\"-> 0.000000000000  , \"mm3\"-> 0.000000000000  , \"T\"->  0.430000000000  , \"B\"-> 12.000000000000  , \"θ\"-> 30.000000000000  |>   , \r\"IDS0298_210427_RAW_cal__sam_\" ->   <| \"ζ\"->  0.028468689077  , \"τ1\"-> 0.020220821810  , \"τS\"-> 0.043529484347  , \"τN\"-> 0.005653540941  , \"τC\"-> 0.003150537442  , \"κ0\"-> 0.000000002855  , \"mm1\"-> 0.000000000000  , \"mm2\"-> 0.000000000000  , \"mm3\"-> 0.000000000000  , \"T\"->  0.430000000000  , \"B\"-> 12.000000000000  , \"θ\"-> 30.000000000000  |>   , \r\"IDS0299_210427_RAW_cal__ref_\" ->   <| \"ζ\"->  0.060257387765  , \"τ1\"-> 0.020933176342  , \"τS\"-> 0.038399909631  , \"τN\"-> 0.009014166994  , \"τC\"-> 0.001999715217  , \"κ0\"-> 0.000000002125  , \"mm1\"-> 0.000000000000  , \"mm2\"-> 0.000000000000  , \"mm3\"-> 0.000000000000  , \"T\"->  0.360000000000  , \"B\"-> 12.000000000000  , \"θ\"-> 30.000000000000  |>   , \r\"IDS0299_210427_RAW_cal__sam_\" ->   <| \"ζ\"->  0.036420486357  , \"τ1\"-> 0.020986681106  , \"τS\"-> 0.049149577509  , \"τN\"-> 0.011109585503  , \"τC\"-> 0.002819780093  , \"κ0\"-> 0.000000002299  , \"mm1\"-> 0.000000000000  , \"mm2\"-> 0.000000000000  , \"mm3\"-> 0.000000000000  , \"T\"->  0.360000000000  , \"B\"-> 12.000000000000  , \"θ\"-> 30.000000000000  |>   , \r\"IDS0300_210427_RAW_cal__ref_\" ->   <| \"ζ\"->  0.338385515343  , \"τ1\"-> 0.049005471612  , \"τS\"-> 0.154718584573  , \"τN\"-> 0.405362096342  , \"τC\"-> 0.001218418583  , \"κ0\"-> 0.000000000425  , \"mm1\"-> 0.000000000000  , \"mm2\"-> 0.000000000000  , \"mm3\"-> 0.000000000000  , \"T\"->  0.140000000000  , \"B\"-> 12.000000000000  , \"θ\"-> 30.000000000000  |>   , \r\"IDS0300_210427_RAW_cal__sam_\" ->   <| \"ζ\"->  0.211545693132  , \"τ1\"-> 0.029106147473  , \"τS\"-> 0.094475691604  , \"τN\"-> 0.369151052631  , \"τC\"-> 0.001396700790  , \"κ0\"-> 0.000000000537  , \"mm1\"-> 0.000000000000  , \"mm2\"-> 0.000000000000  , \"mm3\"-> 0.000000000000  , \"T\"->  0.140000000000  , \"B\"-> 12.000000000000  , \"θ\"-> 30.000000000000  |>   , \r\"IDS0301_210831_RAW_cal__ref_\" ->   <| \"ζ\"->  0.083856390991  , \"τ1\"-> 0.023882632275  , \"τS\"-> 0.042264558819  , \"τN\"-> 0.014926022610  , \"τC\"-> 0.001493479414  , \"κ0\"-> 0.000000001739  , \"mm1\"-> 0.000000000000  , \"mm2\"-> 0.000000000000  , \"mm3\"-> 0.000000000000  , \"T\"->  0.300000000000  , \"B\"-> 12.000000000000  , \"θ\"-> 30.000000000000  |>   , \r\"IDS0301_210831_RAW_cal__sam_\" ->   <| \"ζ\"->  0.050663808076  , \"τ1\"-> 0.024940898568  , \"τS\"-> 0.056803871413  , \"τN\"-> 0.018856862265  , \"τC\"-> 0.002133501904  , \"κ0\"-> 0.000000001888  , \"mm1\"-> 0.000000000000  , \"mm2\"-> 0.000000000000  , \"mm3\"-> 0.000000000000  , \"T\"->  0.300000000000  , \"B\"-> 12.000000000000  , \"θ\"-> 30.000000000000  |>   , \r\"IDS0302_210831_RAW_cal__ref_\" ->   <| \"ζ\"->  0.118191658932  , \"τ1\"-> 0.027786613255  , \"τS\"-> 0.049841575379  , \"τN\"-> 0.030683320319  , \"τC\"-> 0.001300754197  , \"κ0\"-> 0.000000001363  , \"mm1\"-> 0.000000000000  , \"mm2\"-> 0.000000000000  , \"mm3\"-> 0.000000000000  , \"T\"->  0.250000000000  , 
